vi "affichage d'un signal aléatoire.vi"() -> ()   [LabVIEW 2014]
uses:
  <vilib>/measure/NI_MABase.lvlib
panel:
  in  "frequence":dbl(knob) scale=0.0..100.0
  in  "stop":bool
  out "Waveform Chart":waveform(dbl)(graph)
  in  "periode s":dbl(knob) scale=0.0..10.0
  in  "Button Rotatif":dbl(knob) scale=0.0..100.0
  # "affichage d'un signal aléatoire"
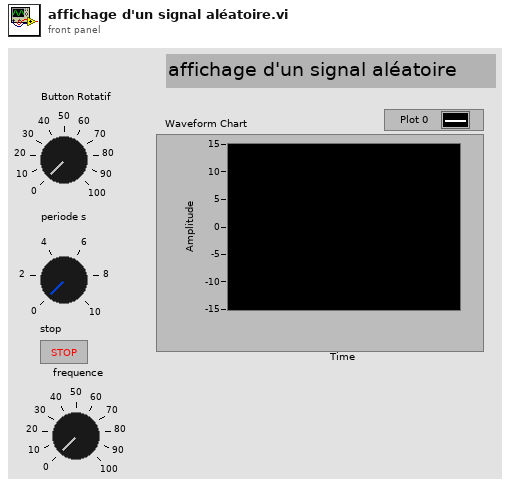
[diagram p1: front panel]
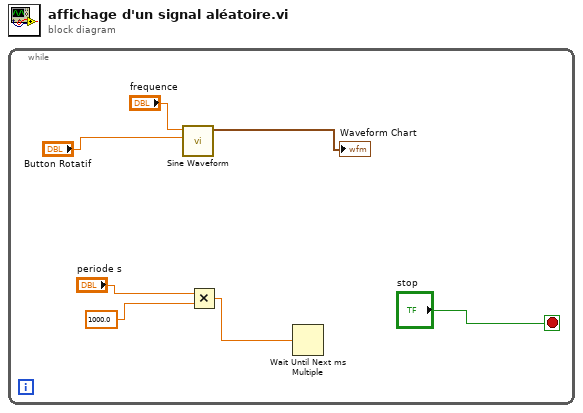
[diagram p0: block diagram]
diagram:
  n1 = while {
    stop <- "stop" stop-if-true
    n2 = call <vilib>:"Sine Waveform.vi"("amplitude"="Button Rotatif", "frequency"="frequence") -> ("signal out"=→"Waveform Chart":waveform(dbl))  [unwired: 8 in, 1 out]
    n3 = Multiply(x="periode s", y=1000.0) -> (x*y=w5:dbl)
    n4 = Wait Until Next ms Multiple(millisecond multiple=w5) -> ()  [unwired: 1 out]
  }
